vi "Create Pattern Script - Rd Capture Frame.vi"(8 "error in (no error)":errorcluster, 10 "FRM Data":T1 {"Addr" format="%x"; "Data" format="%x"}, 11 "SPI 3W Pattern Creator in":refnum<class "SPI 3W Pattern Creator.lvclass">) -> (0 "error out":errorcluster, 2 "String":string, 3 "SPI 3W Pattern Creator out":refnum<class "SPI 3W Pattern Creator.lvclass">)   [LabVIEW 2018, in "SPI 3W Pattern Creator.lvlib" / "SPI 3W Pattern Creator.lvclass"]
uses:
  SPI 3W Pattern Creator.lvclass
  Ctls/Frame Data - SPI_3W.ctl
  Ctls/RW Options.ctl
  Interfaces/Protocol Interface.lvlibp/Interfaces/Protocol Interface/Pin State.ctl
  Protocols/SPI Root Pattern Creator.lvlibp/Plugins/SouceCode/SPI_Pattern Creator/SPI Root/Data Type.ctl
  Protocols/SPI Root Pattern Creator.lvlibp/Plugins/SouceCode/SPI_Pattern Creator/SPI Root/Special Frame Type.ctl
  Interfaces/Protocol Interface.lvlibp/Interfaces/Protocol Interface/Protocol Interface.lvclass
  Protocols/SPI Root Pattern Creator.lvlibp/Plugins/SouceCode/SPI_Pattern Creator/SPI Root/SPI Root Pattern Creator.lvclass
  C:/P4 Workspace/PC Client/Solutions/5g_eap/trunk/1.0/HiSi5GmmWave/Pattern_Gen_Tool/Plugins/Protocols/SPI Root Pattern Creator.lvlibp/Plugins/SouceCode/SPI_Pattern Creator/SPI Root/SPI Root Pattern Creator.lvclass
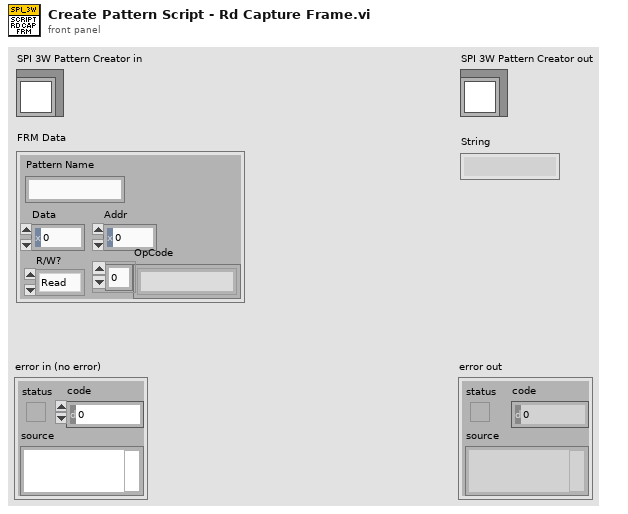
[diagram p1: front panel]
types:
  T1 = typedef "Frame Data - SPI_3W.ctl" = cluster{"Pattern Name":string, "Data":u16, "Addr":u16, "OpCode":string[], "R/W?":T2}
  T2 = typedef "RW Options.ctl" = enum16{"Read", "Write", "R/W"}
  T3 = typedef "SPI Root Pattern Creator.lvlibp/SPI Root Pattern Creator.lvclass/Special Frame Type.ctl" = enum16{"SPI 4W FRM Start", "SPI 4W Wait", "SPI 4W FRM End", "SPI 4W Write Cmd", "SPI Rd Collect Cmd", "SPI Rd Value Cmd", "SPI 3W FRM Start", "SPI 3W Write Cmd", "SPI 3W FRM End", "SPI 3W Wait", "SPI 3W Rd Cmd"}
  T4 = typedef "SPI Root Pattern Creator.lvlibp/SPI Root Pattern Creator.lvclass/Data Type.ctl" = enum16{"Drive", "Compare", "Read"}
  T5 = typedef "Protocol Interface.lvlibp/Protocol Interface.lvclass/Pin State.ctl" = enum16{"0", "1", "L", "H", "X", "V", "D", "M"}
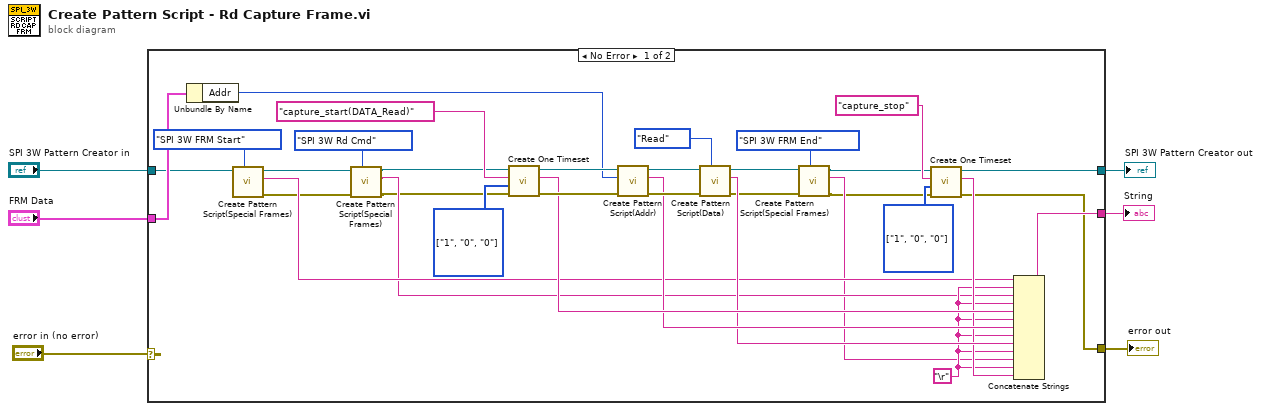
[diagram p0: block diagram]
diagram:
  n1 = case shown="No Error" "error in (no error)" {
    selector: "error in (no error)" -> [_ w41]
    tunnel: "SPI 3W Pattern Creator in" -> [w22 w42]
    tunnel: "FRM Data" -> [w36 _]
    tunnel: [w25 _] -> w3
    tunnel: [w24 w41] -> w2
    tunnel: [w23 w42] -> w1
    frame No Error {
      w26 = "\r"
      w32 = T5[] [enum."1", enum."0", enum."0"] items=["0", "1", "L", "H", "X", "V", "D", "M"] ("PinStates")
      w40 = T5[] [enum."1", enum."0", enum."0"] items=["0", "1", "L", "H", "X", "V", "D", "M"] ("PinStates")
      n2 = Unbundle By Name(w36) -> ("Addr"=w35:u16)
      n3 = call "Create Pattern Script(Special Frames).vi"("Special Frame Type"=Special_Frame_Type."SPI 3W FRM Start", "SPI Root Pattern Creator in"=w22) -> ("error out"=w20:errorcluster, "String out"=w21:string, "SPI Root Pattern Creator out"=w19:refnum<class "SPI 3W Pattern Creator.lvclass">)  [unwired: 7 in]
      n4 = call "Create Pattern Script(Special Frames).vi"("Special Frame Type"=Special_Frame_Type."SPI 3W Rd Cmd", "error in (no error)"=w20, "SPI Root Pattern Creator in"=w19) -> ("error out"=w16:errorcluster, "String out"=w17:string, "SPI Root Pattern Creator out"=w18:refnum<class "SPI 3W Pattern Creator.lvclass">)  [unwired: 6 in]
      n5 = call-dynamic "Create One Timeset.vi"("error in (no error)"=w16, "PinStates"=w40, "OpCode"="capture_start(DATA_Read)", "SPI 3W Pattern Creator in"=w18) -> ("error out"=w38:errorcluster, "String  out"=w30:string, "SPI 3W Pattern Creator out"=w37:refnum<class "SPI 3W Pattern Creator.lvclass">)  [unwired: 5 in]
      n6 = call-dynamic "Create Pattern Script(Addr).vi"("error in (no error)"=w38, "Addr"=w35, "SPI 3W Pattern Creator in"=w37) -> ("error out"=w33:errorcluster, "String"=w29:string, "SPI 3W Pattern Creator out"=w34:refnum<class "SPI 3W Pattern Creator.lvclass">)  [unwired: 6 in]
      n7 = call-dynamic "Create Pattern Script(Data).vi"("Data Type"=Data_Type."Read", "error in (no error)"=w33, "SPI 3W Pattern Creator in"=w34) -> ("error out"=w15:errorcluster, "String"=w28:string, "SPI 3W Pattern Creator out"=w14:refnum<class "SPI 3W Pattern Creator.lvclass">)  [unwired: 6 in]
      n8 = call "Create Pattern Script(Special Frames).vi"("Special Frame Type"=Special_Frame_Type."SPI 3W FRM End", "error in (no error)"=w15, "SPI Root Pattern Creator in"=w14) -> ("error out"=w11:errorcluster, "String out"=w12:string, "SPI Root Pattern Creator out"=w13:refnum<class "SPI 3W Pattern Creator.lvclass">)  [unwired: 6 in]
      n9 = call-dynamic "Create One Timeset.vi"("error in (no error)"=w11, "PinStates"=w32, "OpCode"="capture_stop", "SPI 3W Pattern Creator in"=w13) -> ("error out"=w24:errorcluster, "String  out"=w27:string, "SPI 3W Pattern Creator out"=w23:refnum<class "SPI 3W Pattern Creator.lvclass">)  [unwired: 5 in]
      n10 = Concatenate Strings(w21, w26, w17, w26, w30, w26, w29, w26, w28, w26, w12, w26, w27) -> (w25:string)
    }
    frame Error {
    }
  }
  "error out" <- w2
  "SPI 3W Pattern Creator out" <- w1
  "String" <- w3
